vi "Emballage_BDD_flatprop_table_Liaison.vi"(8 "entrée d'erreur (pas d'erreur)":errorcluster, 9 "NUM_EMBASE":string, 10 "Table_BDD":string, 11 "Champ_resultat":string) -> (0 "sortie d'erreur":errorcluster, 2 "NO_VALVE":string, 3 "données":string[][](array[string]))   [LabVIEW 2020]
uses:
  Modules/FS/60_FS_Controles/60_FS_SetGet.ctl
  <vilib>/addons/database/Connection.llb/DB Tools Open Connec (Path).vi
  <vilib>/addons/database/Connection.llb/Conn Execute.vi
  <vilib>/addons/database/Recordset.llb/Rec Fetch Recordset Data (R).vi
  <vilib>/addons/database/Recordset.llb/Rec Destroy - Connection.vi
  <vilib>/addons/database/NI_Database_API.lvlib
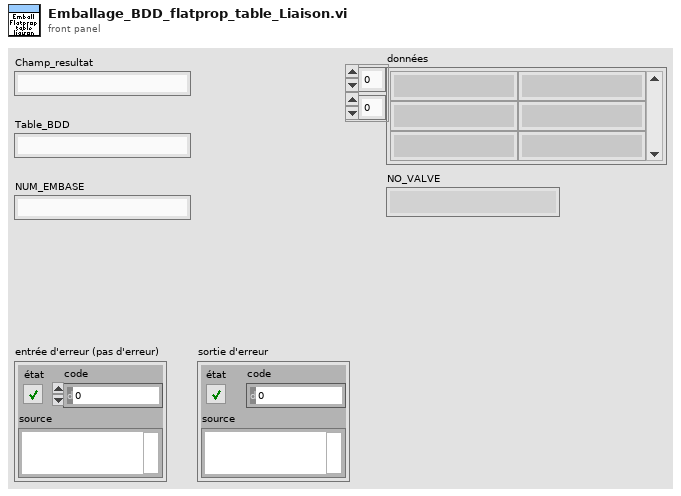
[diagram p1: front panel]
types:
  T1 = typedef "60_FS_SetGet.ctl" = enum16{"set", "get"}
  T2 = typedef "60_FS_CLT_Chemins.ctl" = cluster{"Racine_local":path, "Racine_reseau":path, "Racine_Support_Application":path, "Fichier_Journalisation":path, "Connexion_BDD_VSX":path, "Connexion_BDD_PLZ":path}
  T3 = typedef "NI_Database_API.lvlib/Conn ObjectReference.ctl" = refnum<k1>
  T4 = typedef "NI_Database_API.lvlib/Rec ObjectReference.ctl" = refnum<k1>
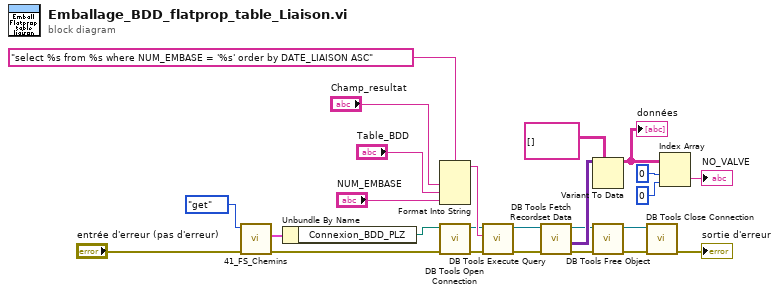
[diagram p0: block diagram]
diagram:
  n1 = call "41_FS_Chemins.vi"("error in (no error)"="entrée d'erreur (pas d'erreur)", "SetGet"=60_FS_SetGet."get") -> ("error out"=w23:errorcluster, "CLT_Chemins_out"=w17:T2)  [unwired: 8 in]
  n2 = Unbundle By Name(w17) -> ("Connexion_BDD_PLZ"=w19:path)
  n3 = Format Into String(format string="select %s from %s where NUM_EMBASE = '%s' order by DATE_LIAISON ASC" ("chaîne de format"), "Champ_resultat", "Table_BDD", "NUM_EMBASE") -> (resulting string=w12:string)  [unwired: 2 in, 1 out]
  n4 = call-poly <vilib>:"DB Tools Open Connection.vi"("error in (no error)"=w23, "connection information"=w19) -> ("error out"=w2:errorcluster, "connection reference"=w1:T3)  [unwired: 6 in]
  n5 = call-poly <vilib>:"DB Tools Execute Query.vi"("error in (no error)"=w2, "SQL query"=w12, "connection reference"=w1) -> ("error out"=w5:errorcluster, "recordset reference"=w7:T4)  [unwired: 5 in]
  n6 = call-poly <vilib>:"DB Tools Fetch Recordset Data.vi"("error in (no error)"=w5, "recordset reference"=w7) -> ("error out"=w6:errorcluster, "recordset data"=w9:variant[][], "recordset reference out"=w8:T4)  [unwired: 3 in]
  n7 = Variant To Data(type=string[][] [], Variant=w9) -> (data=w13:string[][])  [unwired: 1 in, 1 out]
  "données" <- w13
  n8 = call-poly <vilib>:"DB Tools Free Object.vi"("error in (no error)"=w6, "recordset reference"=w8) -> ("error out"=w3:errorcluster, "connection reference"=w4:T3)  [unwired: 8 in]
  n9 = call <vilib>:"DB Tools Close Connection.vi"("error in (no error)"=w3, "connection reference"=w4) -> ("error out"=→"sortie d'erreur":errorcluster)  [unwired: 5 in]
  n10 = Index Array(array=w13, index (row)=0 ("indice (ligne)"), index (col)=0 ("indice désactivé (col)")) -> (element=→"NO_VALVE":string)
